vi "EXAMPLE_PARSEFILE.vi"() -> ()   [LabVIEW 2017]
panel:
  in  "Listbox":i32(listbox)
  out "Variant":variant
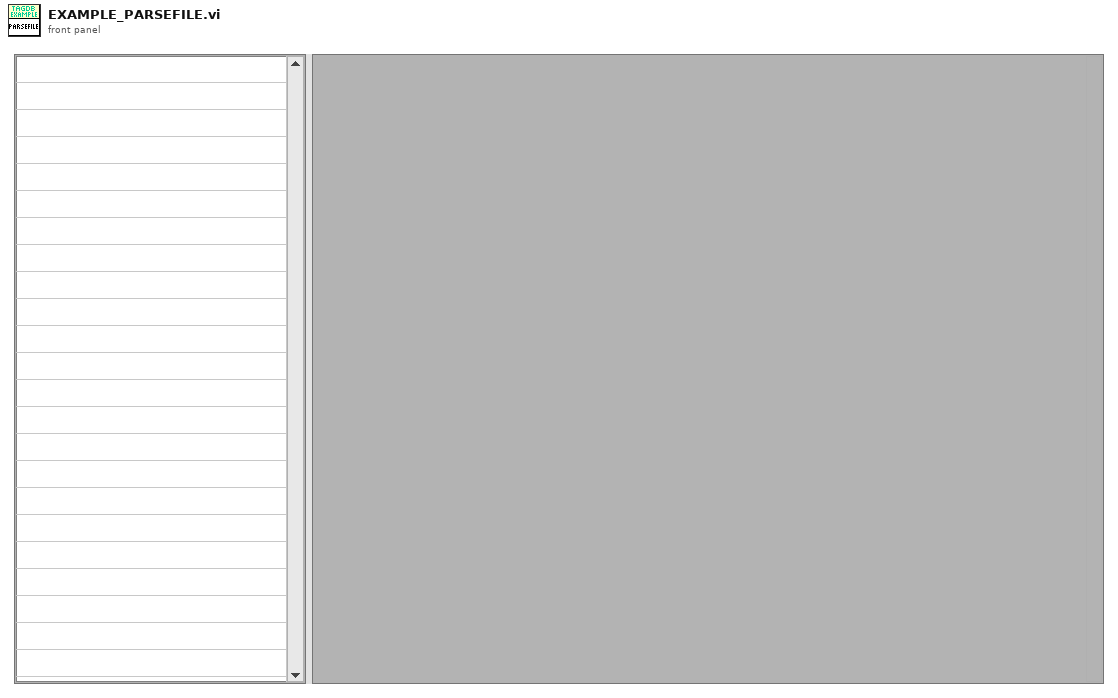
[diagram p1: front panel]
types:
  T1 = enum16{"open", "replace", "create", "open or create", "replace or create", "replace or create with confirmation"}
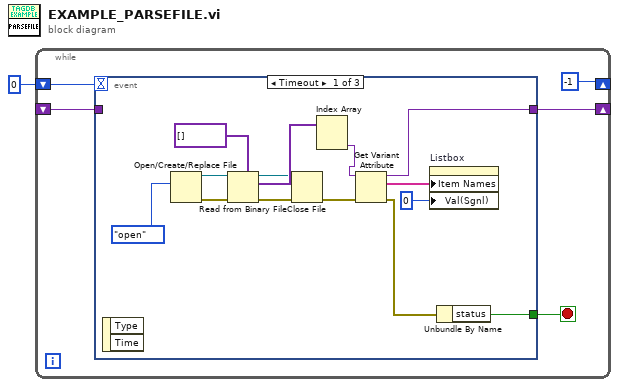
[diagram p0: block diagram]
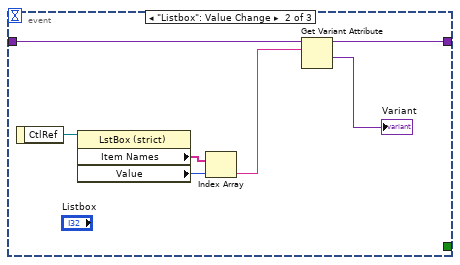
[diagram p2: hidden frame]
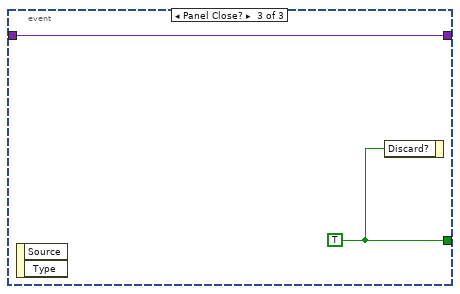
[diagram p3: hidden frame]
diagram:
  n1 = while {
    shift-right: [-1] -> _
    shift-left: 0 -> [w5]
    shift-right: [w3] -> _
    shift-left: _ -> [w2]
    stop <- w6 stop-if-true
    n2 = event shown="[0] Timeout" {
      selector: _ -> [_ _ _]
      dyn-events: _ -> [_ _ _]
      timeout: w5 -> [_ _ _]
      tunnel: [w8 _ w29] -> w6
      tunnel: [w12 w22 w28] -> w3
      tunnel: w2 -> [_ w24 w28]
      event Timeout {
        n3 = event-data() -> ()  [unwired: 1 in, 2 out]
        n4 = Open/Create/Replace File(operation (0:open)=T1."open") -> (refnum out=w15:refnum<file>, error out=w16:errorcluster)  [unwired: 5 in, 1 out]
        n5 = Read from Binary File(5:variant[] [] ("Array"), 8:w16, 11:w15) -> (0:w14:errorcluster, 2:w19:variant[], 3:w13:refnum<file>)  [unwired: 3 in, 1 out]
        n6 = Close File(refnum=w13, error in=w14) -> (error out=w20:errorcluster)  [unwired: 1 out]
        n7 = Index Array(array=w19) -> (element #2=w7:variant)  [unwired: 2 in, 1 out]
        n8 = Get Variant Attribute(Variant=w7, error in=w20) -> (duplicate Variant=w12:variant, names=w11:string[], error out=w9:errorcluster)  [unwired: 2 in, 1 out]
        n9 = property on="Listbox" class="LstBox (strict)"("Item Names"=w11, "Val(Sgnl)"=0 ("Value (Signaling)")) -> ()  [unwired: 2 in, 2 out]
        n10 = Unbundle By Name(w9) -> ("status"=w8:bool)
      }
      event "Listbox": Value Change {
        n11 = event-data() -> ("CtlRef"=w27:refnum<vi>)  [unwired: 1 in]
        n12 = property class="LstBox (strict)"(reference=w27) -> ("Item Names"=w25:string[], "Value"=w26:i32)  [unwired: 1 in, 2 out]
        n13 = Index Array(array=w25, index=w26) -> (element=w23:string)
        n14 = Get Variant Attribute(Variant=w24, name=w23) -> (duplicate Variant=w22:variant, value=→"Variant":variant)  [unwired: 2 in, 2 out]
      }
      event Panel Close? {
        w29 = TRUE
        n15 = event-data() -> ()  [unwired: 1 in, 2 out]
        n16 = event-data("Discard?"=w29) -> ()  [unwired: 1 in, 1 out]
      }
    }
  }
